vi "Validate Tag Settings.vi"(0 "PulseWidth (ms)":dbl, 1 "Minimum file size (s)":dbl=-1.0, 2 "Minimum sample rate (Hz)":dbl=-1.0, 5 "TaggingPeriod (pws)":u32, 9 "Minimum tagging period (pws)":u32, 12 "Minimum tags per file":u32, 14 "Minimum samples per pulse":dbl) -> (4 "Valid":bool, 15 "Info":string)   [LabVIEW 2017]
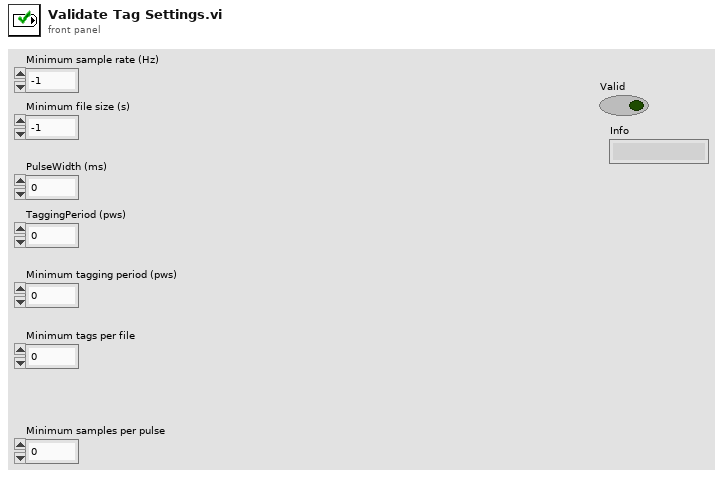
[diagram p1: front panel]
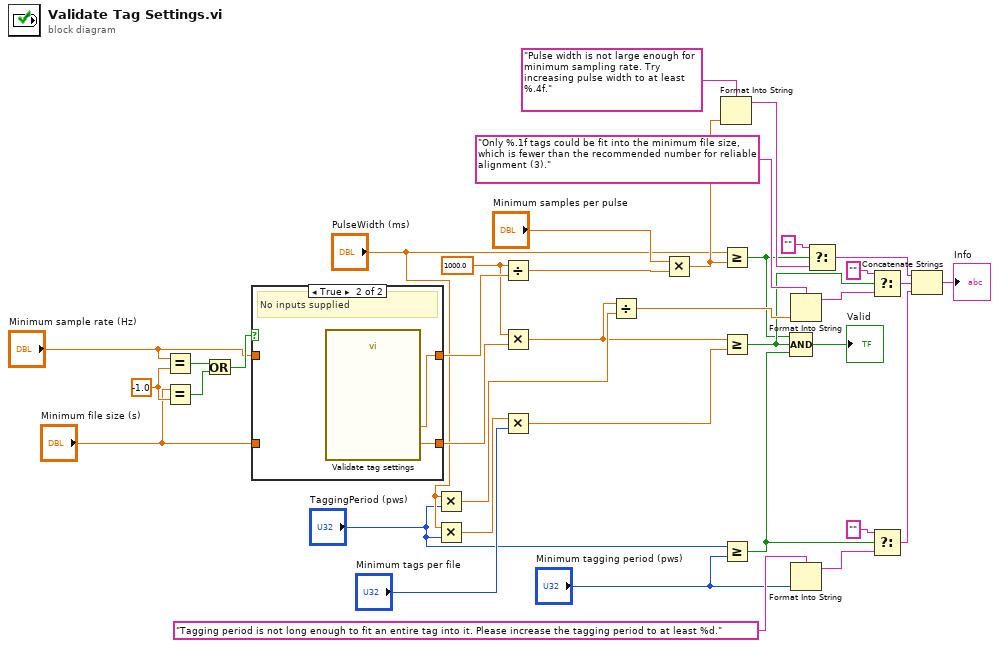
[diagram p0: block diagram]
diagram:
  w8 = -1.0 ("y")
  w13 = 1000.0
  n1 = Equal?(x="Minimum sample rate (Hz)", y=w8) -> (x = y?=w7:bool)
  n2 = Equal?(x="Minimum file size (s)", y=w8) -> (x = y?=w6:bool)
  n3 = Or(x=w7, y=w6) -> (x .or. y?=w5:bool)
  n4 = case shown="True" w5 {
    tunnel: [w40 w42] -> w15
    tunnel: [w39 w41] -> w11
    tunnel: "Minimum sample rate (Hz)" -> [w40 _]
    tunnel: "Minimum file size (s)" -> [w39 _]
    frame False {
    }
    frame True {
      # "No inputs supplied"
      n5 = call "Validate tag settings"() -> ("Minimum file size (s)"=w41:dbl, "Minimum sampling rate (Hz)"=w42:dbl)  [unwired: 16 in, 2 out]
    }
  }
  n6 = Multiply(x="PulseWidth (ms)", y="TaggingPeriod (pws)") -> (x*y=w29:dbl)
  n7 = Multiply(x="PulseWidth (ms)", y="TaggingPeriod (pws)") -> (x*y=w10:dbl)
  n8 = Divide(x=w13, y=w15) -> (x/y=w17:dbl)
  n9 = Multiply(x=w13, y=w11) -> (x*y=w28:dbl)
  n10 = Multiply(x=w10, y="Minimum tags per file") -> (x*y=w12:dbl)
  n11 = Divide(x=w28, y=w29) -> (x/y=w31:dbl)
  n12 = Multiply(x="Minimum samples per pulse", y=w17) -> (x*y=w26:dbl)
  n13 = Format Into String(format string="Pulse width is not large enough for minimum sampling rate. Try increasing pulse width to at least %.4f.", w26) -> (resulting string=w27:string)  [unwired: 2 in, 1 out]
  n14 = Greater Or Equal?(x="PulseWidth (ms)", y=w26) -> (x >= y?=w19:bool)
  n15 = Greater Or Equal?(x=w28, y=w12) -> (x >= y?=w20:bool)
  n16 = Greater Or Equal?(x="TaggingPeriod (pws)", y="Minimum tagging period (pws)") -> (x >= y?=w21:bool)
  n17 = Compound Arithmetic op=AND(w19, w20, w21) -> (→"Valid":bool)
  n18 = Format Into String(format string="Only %.1f tags could be fit into the minimum file size, which is fewer than the recommended number for reliable alignment (3).", w31) -> (resulting string=w32:string)  [unwired: 2 in, 1 out]
  n19 = Format Into String(format string="Tagging period is not long enough to fit an entire tag into it. Please increase the tagging period to at least %d.", "Minimum tagging period (pws)") -> (resulting string=w38:string)  [unwired: 2 in, 1 out]
  n20 = Select(t="", s=w19, f=w27) -> (s? t:f=w33:string)
  n21 = Select(t="", s=w20, f=w32) -> (s? t:f=w34:string)
  n22 = Select(t="", s=w21, f=w38) -> (s? t:f=w35:string)
  n23 = Concatenate Strings(w33, w34, w35) -> (→"Info":string)
